vi "Drive Globals.vi"() -> ()   [LabVIEW 2019]
panel:
  in  "HighGear?":bool
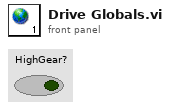
[diagram p1: front panel]
diagram:
